vi "Open and Configure Digital Session.vi"(5 "pin list":string, 7 "waveform name":string, 8 "error in":errorcluster, 10 "Digital pattern folder":path, 11 "Digital resource":refnum<k15>="6571" caption="resource name") -> (0 "error out":errorcluster, 3 "Digital session":refnum<k15>)   [LabVIEW 2021]
uses:
  <instrlib>/niDigital/niDigital.llb/niDigital Bit Order.ctl
  <instrlib>/niDigital/niDigital.llb/niDigital Data Mapping.ctl
  <instrlib>/niDigital/niDigital.llb/niDigital Load Specifications Levels and Timing (Single).vi
  <instrlib>/niDigital/niDigital.llb/niDigital Create Source Waveform (Serial).vi
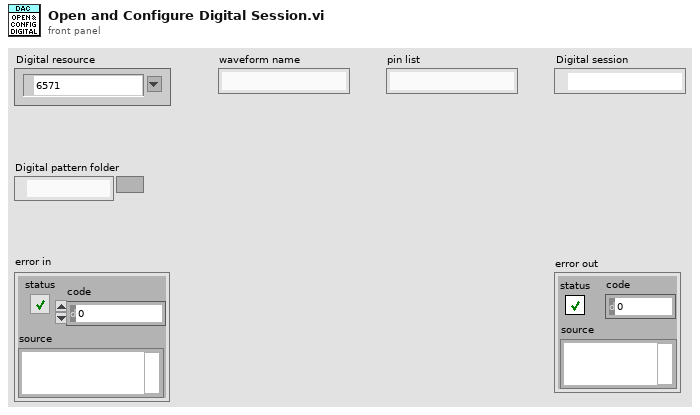
[diagram p1: front panel]
types:
  T1 = typedef "niDigital Data Mapping.ctl" = i32
  T2 = typedef "niDigital Bit Order.ctl" = i32
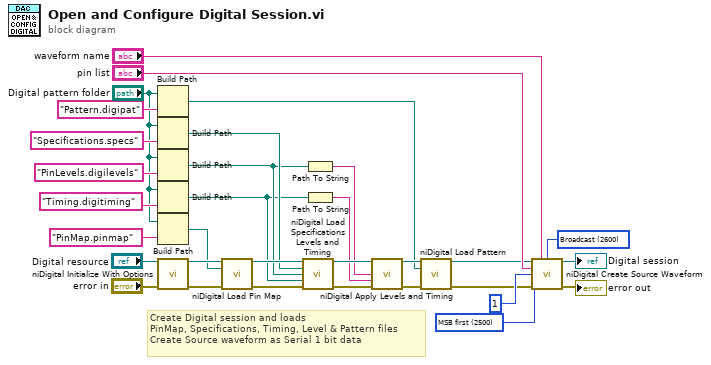
[diagram p0: block diagram]
diagram:
  w5 = T1 2600 items=["Broadcast"=2600, "Site Unique"=2601] ("data mapping")
  w6 = T2 2500 items=["MSB first"=2500, "LSB first"=2501] ("bit order")
  # "Create Digital session and loads\nPinMap, Specifications, Timing, Level & Pattern files\nCreate Source waveform as Serial 1 bit data"
  n1 = Build Path(base path="Digital pattern folder", name or relative path="Pattern.digipat") -> (appended path=w12:path)
  n2 = Build Path(base path="Digital pattern folder", name or relative path="Specifications.specs") -> (appended path=w18:path)
  n3 = Build Path(base path="Digital pattern folder", name or relative path="PinLevels.digilevels") -> (appended path=w16:path)
  n4 = Build Path(base path="Digital pattern folder", name or relative path="Timing.digitiming") -> (appended path=w14:path)
  n5 = Build Path(base path="Digital pattern folder", name or relative path="PinMap.pinmap") -> (appended path=w20:path)
  n6 = call <instrlib>:"niDigital Initialize With Options.vi"("resource name"="Digital resource", "error in"="error in") -> ("instrument handle"=w28:refnum<k15>, "error out"=w27:errorcluster)  [unwired: 12 in]
  n7 = call <instrlib>:"niDigital Load Pin Map.vi"("instrument handle"=w28, "pin map file"=w20, "error in"=w27) -> ("instrument handle out"=w26:refnum<k15>, "error out"=w25:errorcluster)  [unwired: 11 in]
  n8 = call-poly <instrlib>:"niDigital Load Specifications Levels and Timing.vi"("instrument handle"=w26, "specifications file path"=w18, "levels file path"=w16, "timing file path"=w14, "error in"=w25) -> ("instrument handle out"=w32:refnum<k15>, "error out"=w31:errorcluster)  [unwired: 9 in]
  n9 = Path To String(path=w16) -> (string=w24:string)
  n10 = Path To String(path=w14) -> (string=w23:string)
  n11 = call <instrlib>:"niDigital Apply Levels and Timing.vi"("instrument handle"=w32, "levels sheet"=w24, "timing sheet"=w23, "error in"=w31) -> ("instrument handle out"=w29:refnum<k15>, "error out"=w30:errorcluster)  [unwired: 10 in]
  n12 = call <instrlib>:"niDigital Load Pattern.vi"("instrument handle"=w29, "pattern file"=w12, "error in"=w30) -> ("instrument handle out"=w4:refnum<k15>, "error out"=w2:errorcluster)  [unwired: 11 in]
  n13 = call-poly <instrlib>:"niDigital Create Source Waveform.vi"("instrument handle"=w4, "waveform name"="waveform name", "data mapping"=w5, "pin list"="pin list", "sample width"=u32 1, "bit order"=w6, "error in"=w2) -> ("instrument handle out"=→"Digital session":refnum<k15>, "error out"=→"error out":errorcluster)  [unwired: 7 in]
